vi "control_lasers_from_CSV_with_SM2.vi"() -> ()   [LabVIEW 2021]
uses:
  <vilib>/DAQmx/write.llb/DAQmx Write (Analog 1D DBL NChan 1Samp).vi
  <vilib>/DAQmx/create/channels.llb/DAQmx Create Channel (AO-Voltage-Basic).vi
  <vilib>/Utility/file.llb/Read Delimited Spreadsheet (DBL).vi
  <vilib>/DAQmx/configure/timing.llb/DAQmx Timing (Sample Clock).vi
  <vilib>/DAQmx/miscellaneous.llb/DAQmx Fill In Error Info.vi
panel:
  out "Y2":dbl
  out "X2":dbl
  out "Cycles Completed":i32
  out "561 (Automated)":dbl
  out "Phase II Iterations":i32
  in  "TickLength":u32
  in  "Blanking (0-10v)":dbl=10.0
  in  "514 (0-10v)":dbl
  in  "488 (0-10v)":dbl
  in  "445 (0-10v)":dbl
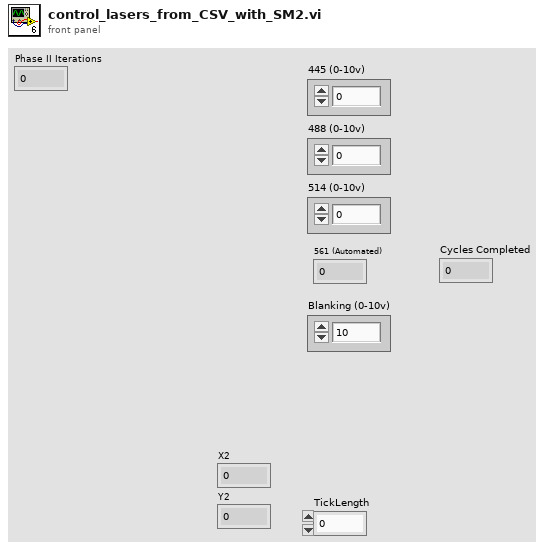
[diagram p1: front panel]
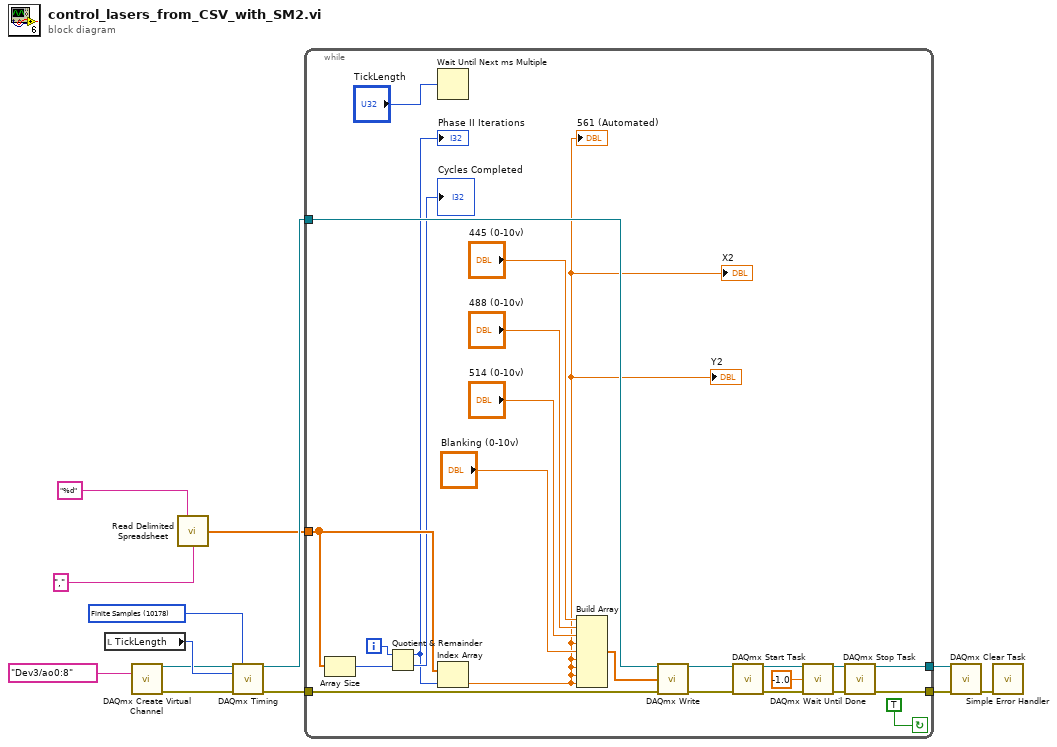
[diagram p0: block diagram]
diagram:
  w11 = 10178 items=["Finite Samples"=10178, "Continuous Samples"=10123, "Hardware Timed Single Point"=12522] ("sample mode")
  n1 = local read "TickLength"() -> (w10:u32)
  n2 = call-poly <vilib>:"DAQmx Create Virtual Channel.vi"("physical channels"=tag "Dev3/ao0:8") -> ("task out"=w7:refnum<k21>, "error out"=w6:errorcluster)  [unwired: 13 in]
  n3 = call-poly <vilib>:"Read Delimited Spreadsheet.vi"("format (%.3f)"="%d", "delimiter (\\t)"=",") -> ("first row"=w1:dbl[])  [unwired: 8 in, 5 out]
  n4 = call-poly <vilib>:"DAQmx Timing.vi"("task/channels in"=w7, "sample mode"=w11, "rate"=w10, "error in"=w6) -> ("task out"=w4:refnum<k21>, "error out"=w5:errorcluster)  [unwired: 10 in]
  n5 = while {
    tunnel: [w25] -> w9
    tunnel: [w26] -> w8
    tunnel: w5 -> [w21]
    tunnel: w4 -> [w20]
    tunnel: w1 -> [w18]
    i -> [w19]
    stop <- TRUE continue-if-true
    n6 = Array Size(array=w18) -> (size(s)=w17:i32)
    n7 = Quotient & Remainder(x=w19, y=w17) -> (x-y*floor(x/y)=w15:i32, floor(x/y)=→"Cycles Completed":i32)
    "Phase II Iterations" <- w15
    n8 = Wait Until Next ms Multiple(millisecond multiple="TickLength") -> ()  [unwired: 1 out]
    n9 = Index Array "Index Array"(array=w18, index=w15) -> (element=w14:dbl)
    "561 (Automated)" <- w14
    "X2" <- w14
    "Y2" <- w14
    n10 = Build Array("445 (0-10v)", "488 (0-10v)", "514 (0-10v)", w14, "Blanking (0-10v)", w14, w14, w14, w14) -> (w37:dbl[])
    n11 = call-poly <vilib>:"DAQmx Write.vi"("task/channels in"=w20, "data"=w37, "error in"=w21) -> ("task out"=w22:refnum<k21>, "error out"=w29:errorcluster)  [unwired: 10 in, 1 out]
    n12 = call <vilib>:"DAQmx Start Task.vi"("task/channels in"=w22, "error in"=w29) -> ("task out"=w23:refnum<k21>, "error out"=w28:errorcluster)  [unwired: 12 in]
    n13 = call <vilib>:"DAQmx Wait Until Done.vi"("task/channels in"=w23, "timeout (sec)"=-1.0, "error in"=w28) -> ("task out"=w24:refnum<k21>, "error out"=w27:errorcluster)  [unwired: 11 in]
    n14 = call <vilib>:"DAQmx Stop Task.vi"("task/channels in"=w24, "error in"=w27) -> ("task out"=w25:refnum<k21>, "error out"=w26:errorcluster)  [unwired: 12 in]
  }
  n15 = call <vilib>:"DAQmx Clear Task.vi"("task in"=w9, "error in"=w8) -> ("error out"=w13:errorcluster)  [unwired: 13 in]
  n16 = call <vilib>:"Simple Error Handler.vi"("error in (no error)"=w13) -> ()  [unwired: 4 in, 5 out]
